vi "Fric Compensator.vi"(10 "Static Friction Voltage":dbl, 11 "Voltage Commands":dbl[](array[numeric])) -> (3 "Friction Compesated Voltage":dbl[](array[numeric]))   [LabVIEW 2017]
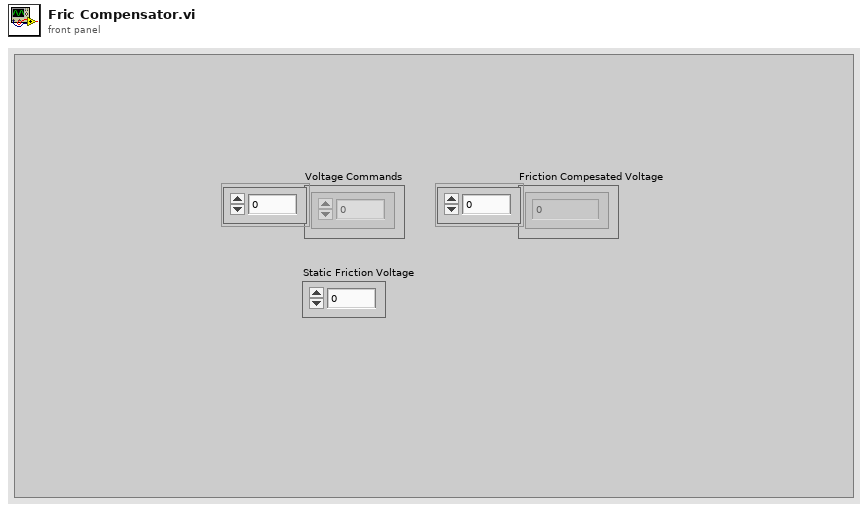
[diagram p1: front panel]
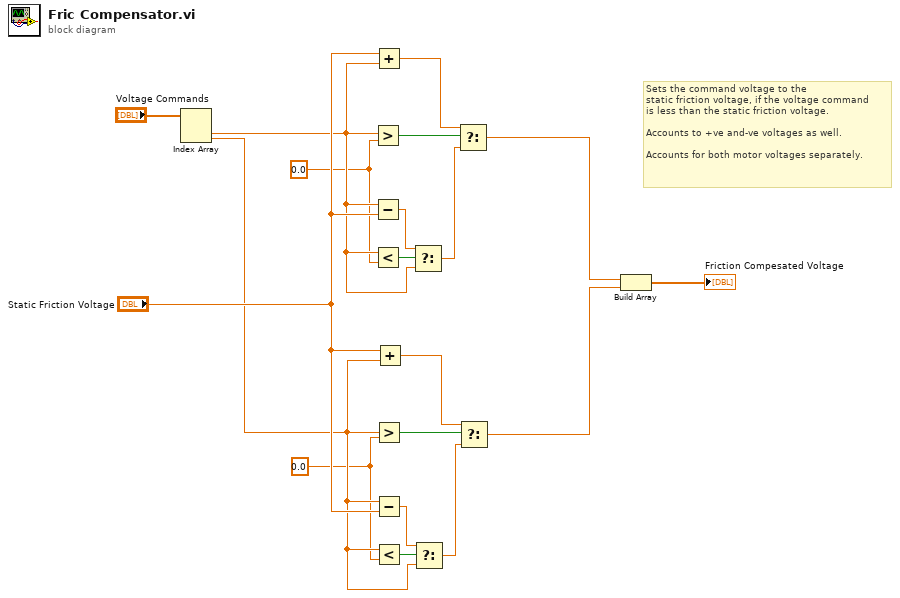
[diagram p0: block diagram]
diagram:
  w10 = 0.0 ("y")
  w3 = 0.0 ("y")
  # "Sets the command voltage to the \nstatic friction voltage, if the voltage command\nis less than the static friction voltage. \n\nAccounts to +ve and-ve voltages as well.\n\nAccounts for both motor voltages separately."
  n1 = Index Array(array="Voltage Commands") -> (element #1=w8:dbl, element #2=w15:dbl)  [unwired: 2 in]
  n2 = Greater?(x=w8, y=w3) -> (0:w2:bool)
  n3 = Subtract(x=w8, y="Static Friction Voltage") -> (x-y=w6:dbl)
  n4 = Less?(x=w8, y=w3) -> (x < y?=w4:bool)
  n5 = Add(x="Static Friction Voltage", y=w8) -> (x+y=w5:dbl)
  n6 = Greater?(x=w15, y=w10) -> (0:w9:bool)
  n7 = Subtract(x=w15, y="Static Friction Voltage") -> (x-y=w13:dbl)
  n8 = Less?(x=w15, y=w10) -> (x < y?=w11:bool)
  n9 = Add(x="Static Friction Voltage", y=w15) -> (x+y=w12:dbl)
  n10 = Select(t=w6, s=w4, f=w8) -> (s? t:f=w7:dbl)
  n11 = Select(t=w13, s=w11, f=w15) -> (s? t:f=w14:dbl)
  n12 = Select(t=w5, s=w2, f=w7) -> (s? t:f=w17:dbl)
  n13 = Select(t=w12, s=w9, f=w14) -> (s? t:f=w18:dbl)
  n14 = Build Array(w17, w18) -> (→"Friction Compesated Voltage":dbl[])
